vi "Release.vi"(8 "error in (no error)":errorcluster, 11 "Panel Control Counter in":refnum<class "Panel Control Counter.lvclass">) -> (0 "error out":errorcluster, 2 "Fully Released?":bool)   [LabVIEW 2023, in "Panel Actor.lvlib" / "Panel.lvlib" / "Panel Control Counter.lvclass"]
doc: "Releases the current Control Counter.\n\n----\nPlease see the following web address for additional documentation and tutorial information:\nhttp://www.mooregoodideas.com/mgi-panel-manager/\n\nAuthor: Derek Trepanier\n\nCopyright (c) 2018, Moore Good Ideas, Inc.\n\nAll rights reserved.\n\nRedistribution and use in source and binary forms, with or without modification, are permitted provided that the following conditions are met:\n\n * Redistributions of source code must retain the above copyright notice, this list of conditions and the following disclaimer.\n * Redistributions in binary form must reproduce the above copyright notice, this list of conditions and the following disclaimer in the documentation and/or other materials provided with the distribution.\n * Neither the name of Moore Good Ideas, Inc. nor the names of its contributors may be used to endorse or promote products derived from this software without specific prior written permission.\n\nTHIS SOFTWARE IS PROVIDED BY THE COPYRIGHT HOLDERS AND CONTRIBUTORS \"AS IS\" AND ANY EXPRESS OR IMPLIED WARRANTIES, INCLUDING, BUT NOT LIMITED TO, THE IMPLIED WARRANTIES OF MERCHANTABILITY AND FITNESS FOR A PARTICULAR PURPOSE ARE DISCLAIMED. IN NO EVENT SHALL THE COPYRIGHT OWNER OR CONTRIBUTORS BE LIABLE FOR ANY DIRECT, INDIRECT, INCIDENTAL, SPECIAL, EXEMPLARY, OR CONSEQUENTIAL DAMAGES (INCLUDING, BUT NOT LIMITED TO, PROCUREMENT OF SUBSTITUTE GOODS OR SERVICES; LOSS OF USE, DATA, OR PROFITS; OR BUSINESS INTERRUPTION) HOWEVER CAUSED AND ON ANY THEORY OF LIABILITY, WHETHER IN CONTRACT, STRICT LIABILITY, OR TORT (INCLUDING NEGLIGENCE OR OTHERWISE) ARISING IN ANY WAY OUT OF THE USE OF THIS SOFTWARE, EVEN IF ADVISED OF THE POSSIBILITY OF SUCH DAMAGE."
uses:
  Panel Control Counter.lvclass
  Panel Control Counter.lvclass/Panel Control Counter.ctl
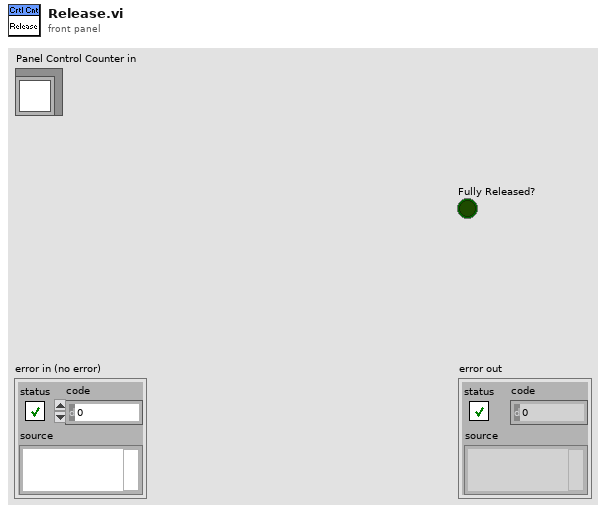
[diagram p1: front panel]
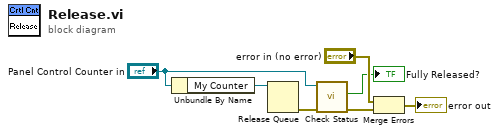
[diagram p0: block diagram]
diagram:
  n1 = Unbundle By Name("Panel Control Counter in") -> ("My Counter"=w6:refnum<queue>)
  n2 = Release Queue(queue=w6) -> (error out=w4:errorcluster)  [unwired: 2 in, 2 out]
  n3 = call "Check Status.vi"("error in (no error)"=w4, "Panel Control Counter in"="Panel Control Counter in") -> ("error out"=w3:errorcluster, "Fully Released?"=→"Fully Released?":bool)  [unwired: 8 in]
  n4 = Merge Errors("error in (no error)", w3) -> (→"error out":errorcluster)
